vi "Unflatten.vi"(8 "error in (no error)":errorcluster, 11 "Pulse Gen Basic Scan in":refnum<class "Pulse Gen Basic Scan.lvclass">) -> (0 "error out":errorcluster, 3 "Pulse Gen Basic Scan out":refnum<class "Pulse Gen Basic Scan.lvclass">)   [LabVIEW 2017, in "Pulse Gen Basic Scan.lvclass"]
uses:
  Pulse Gen Basic Scan.lvclass
  Pulse Gen Basic Scan.lvclass/Pulse Gen Basic Scan.ctl
  Global/File Locations.vi
  Scanner/Scanner.lvclass
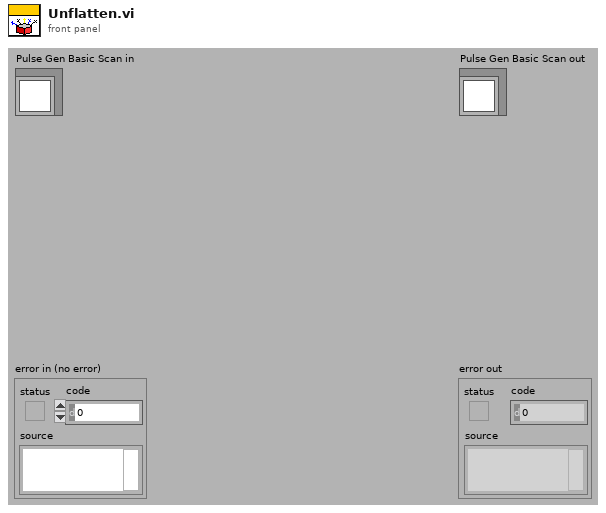
[diagram p1: front panel]
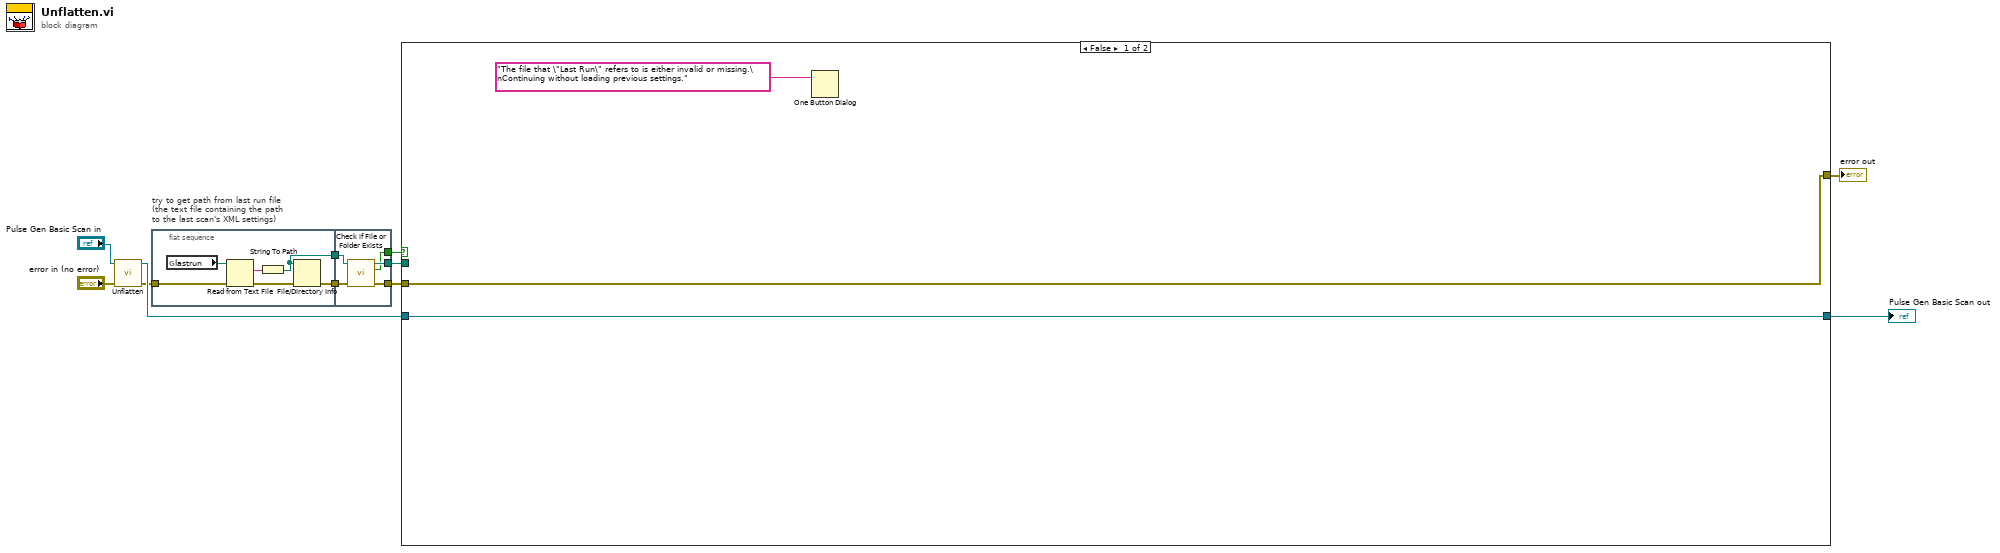
[diagram p0: block diagram]
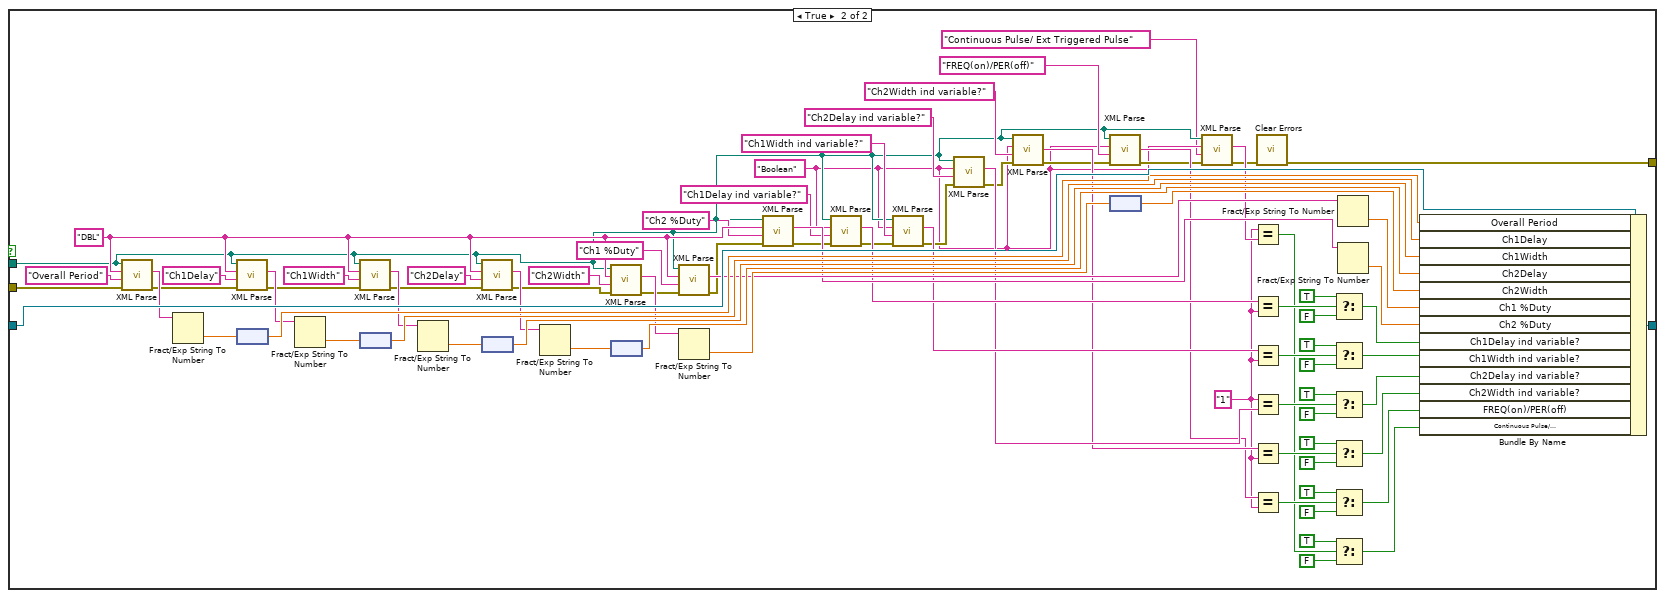
[diagram p2: hidden frame]
diagram:
  n1 = call-parent "Unflatten.vi"("error in (no error)"="error in (no error)", "Scanner in"="Pulse Gen Basic Scan in") -> ("error out"=w7:errorcluster, "Scanner out"=w11:refnum<class "Pulse Gen Basic Scan.lvclass">)  [unwired: 8 in]
  n2 = flat-sequence "try to get path from last run file\n(the text file containing the path\nto the last scan's XML settings)" {
    tunnel: w7 -> [w12]
    tunnel: [w17] -> w4
    tunnel: [w13] -> w3
    tunnel: [w21] -> w6
    tunnel: [w19] -> w5
    tunnel: w4 -> [w20]
    tunnel: w3 -> [w22]
    tunnel: [w18] -> w2
    frame #0 {
      n3 = global read "File Locations.vi" "lastrun"() -> (w15:path)
      n4 = Read from Text File(file (use dialog)=w15, error in=w12) -> (text=w16:string, error out=w14:errorcluster)  [unwired: 4 out]
      n5 = String To Path(string=w16) -> (path=w17:path)
      n6 = File/Directory Info(path=w17, error in=w14) -> (error out=w13:errorcluster)  [unwired: 6 out]
    }
    frame #1 {
      n7 = call <vilib>:"Check if File or Folder Exists.vi"("error in (no error)"=w22, "path"=w20) -> ("error out"=w21:errorcluster, "file or folder exists?"=w18:bool, "dup path"=w19:path)  [unwired: 7 in]
    }
  }
  n8 = case shown="False" w2 {
    tunnel: w11 -> [w25 w108]
    tunnel: [w25 w107] -> w8
    tunnel: w6 -> [w23 w105]
    tunnel: w5 -> [_ w29]
    tunnel: [w23 w26] -> w1
    frame False {
      n9 = One Button Dialog(message="The file that \"Last Run\" refers to is either invalid or missing.\nContinuing without loading previous settings.") -> ()  [unwired: 1 in, 1 out]
    }
    frame True {
      w32 = "1"
      w28 = "Boolean"
      w77 = "DBL"
      n10 = call "XML Parse.vi"("error in (no error)"=w105, "Name String"="Overall Period", "Type String"=w77, "Path"=w29) -> ("error out"=w101:errorcluster, "String Out"=w104:string)  [unwired: 6 in]
      n11 = Fract/Exp String To Number(string=w104) -> (number=w103:dbl)  [unwired: 3 in, 1 out]
      n12 = call "XML Parse.vi"("error in (no error)"=w101, "Name String"="Ch1Delay", "Type String"=w77, "Path"=w29) -> ("error out"=w96:errorcluster, "String Out"=w99:string)  [unwired: 6 in]
      n13 = node(w103) -> (w102:dbl[unit])
      n14 = Fract/Exp String To Number(string=w99) -> (number=w98:dbl)  [unwired: 3 in, 1 out]
      n15 = call "XML Parse.vi"("error in (no error)"=w96, "Name String"="Ch1Width", "Type String"=w77, "Path"=w29) -> ("error out"=w90:errorcluster, "String Out"=w94:string)  [unwired: 6 in]
      n16 = node(w98) -> (w97:dbl[unit])
      n17 = Fract/Exp String To Number(string=w94) -> (number=w93:dbl)  [unwired: 3 in, 1 out]
      n18 = call "XML Parse.vi"("error in (no error)"=w90, "Name String"="Ch2Delay", "Type String"=w77, "Path"=w29) -> ("error out"=w86:errorcluster, "String Out"=w87:string)  [unwired: 6 in]
      n19 = node(w93) -> (w92:dbl[unit])
      n20 = Fract/Exp String To Number(string=w87) -> (number=w88:dbl)  [unwired: 3 in, 1 out]
      n21 = call "XML Parse.vi"("error in (no error)"=w86, "Name String"="Ch2Width", "Type String"=w77, "Path"=w29) -> ("error out"=w81:errorcluster, "String Out"=w84:string)  [unwired: 6 in]
      n22 = node(w88) -> (w89:dbl[unit])
      n23 = call "XML Parse.vi"("error in (no error)"=w81, "Name String"="Ch1 %Duty", "Type String"=w77, "Path"=w29) -> ("error out"=w75:errorcluster, "String Out"=w79:string)  [unwired: 6 in]
      n24 = Fract/Exp String To Number(string=w84) -> (number=w83:dbl)  [unwired: 3 in, 1 out]
      n25 = call "XML Parse.vi"("error in (no error)"=w75, "Name String"="Ch2 %Duty", "Type String"=w77, "Path"=w29) -> ("error out"=w71:errorcluster, "String Out"=w74:string)  [unwired: 6 in]
      n26 = call "XML Parse.vi"("error in (no error)"=w71, "Name String"="Ch1Delay ind variable?", "Type String"=w28, "Path"=w29) -> ("error out"=w64:errorcluster, "String Out"=w70:string)  [unwired: 6 in]
      n27 = call "XML Parse.vi"("error in (no error)"=w64, "Name String"="Ch1Width ind variable?", "Type String"=w28, "Path"=w29) -> ("error out"=w58:errorcluster, "String Out"=w60:string)  [unwired: 6 in]
      n28 = call "XML Parse.vi"("error in (no error)"=w58, "Name String"="Ch2Delay ind variable?", "Type String"=w28, "Path"=w29) -> ("error out"=w51:errorcluster, "String Out"=w54:string)  [unwired: 6 in]
      n29 = call "XML Parse.vi"("error in (no error)"=w51, "Name String"="Ch2Width ind variable?", "Type String"=w28, "Path"=w29) -> ("error out"=w43:errorcluster, "String Out"=w47:string)  [unwired: 6 in]
      n30 = call "XML Parse.vi"("error in (no error)"=w43, "Name String"="FREQ(on)/PER(off)", "Type String"=w28, "Path"=w29) -> ("error out"=w31:errorcluster, "String Out"=w38:string)  [unwired: 6 in]
      n31 = node(w83) -> (w82:dbl[unit])
      n32 = call "XML Parse.vi"("error in (no error)"=w31, "Name String"="Continuous Pulse/ Ext Triggered Pulse", "Type String"=w28, "Path"=w29) -> ("error out"=w30:errorcluster, "String Out"=w33:string)  [unwired: 6 in]
      n33 = Equal?(x=w32, y=w33) -> (x = y?=w34:bool)
      n34 = Equal?(x=w70, y=w32) -> (x = y?=w69:bool)
      n35 = Equal?(x=w60, y=w32) -> (x = y?=w63:bool)
      n36 = Equal?(x=w32, y=w54) -> (x = y?=w57:bool)
      n37 = Equal?(x=w47, y=w32) -> (x = y?=w50:bool)
      n38 = Equal?(x=w38, y=w32) -> (x = y?=w42:bool)
      n39 = call <vilib>:"Clear Errors.vi"("error in (no error)"=w30) -> ("error out"=w26:errorcluster)  [unwired: 5 in, 1 out]
      n40 = Select(t=TRUE, s=w69, f=FALSE) -> (s? t:f=w66:bool)
      n41 = Select(t=TRUE, s=w63, f=FALSE) -> (s? t:f=w59:bool)
      n42 = Select(t=TRUE, s=w57, f=FALSE) -> (s? t:f=w53:bool)
      n43 = Select(t=TRUE, s=w50, f=FALSE) -> (s? t:f=w46:bool)
      n44 = Select(t=TRUE, s=w42, f=FALSE) -> (s? t:f=w39:bool)
      n45 = Select(t=TRUE, s=w34, f=FALSE) -> (s? t:f=w35:bool)
      n46 = Fract/Exp String To Number(string=w79) -> (number=w78:dbl)  [unwired: 3 in, 1 out]
      n47 = Fract/Exp String To Number(string=w74) -> (number=w73:dbl)  [unwired: 3 in, 1 out]
      n48 = Bundle By Name(cluster=w108, "Overall Period"=w102, "Ch1Delay"=w97, "Ch1Width"=w92, "Ch2Delay"=w89, "Ch2Width"=w82, "Ch1 %Duty"=w78, "Ch2 %Duty"=w73, "Ch1Delay ind variable?"=w66, "Ch1Width ind variable?"=w59, "Ch2Delay ind variable?"=w53, "Ch2Width ind variable?"=w46, "FREQ(on)/PER(off)"=w39, "Continuous Pulse/ \nExt Triggered Pulse"=w35) -> (w107:refnum<class "Pulse Gen Basic Scan.lvclass">)
    }
  }
  "Pulse Gen Basic Scan out" <- w8
  "error out" <- w1
